vi "Day 9 - Rope Bridge.vi"() -> ()   [LabVIEW 2020, in "AoC 2022.lvlib"]
uses:
  AoC 2022.lvlib
panel:
  in  "Puzzle Input":string="R 4\nU 4\nL 3\nD 1\nR 4\nD 1\nL 5\nR 2"
  out "Puzzle Part-2 Answer":string
  out "Puzzle Answer":string
  # "Press Ctrl+M & Enter the Puzzle Input and run the VI"
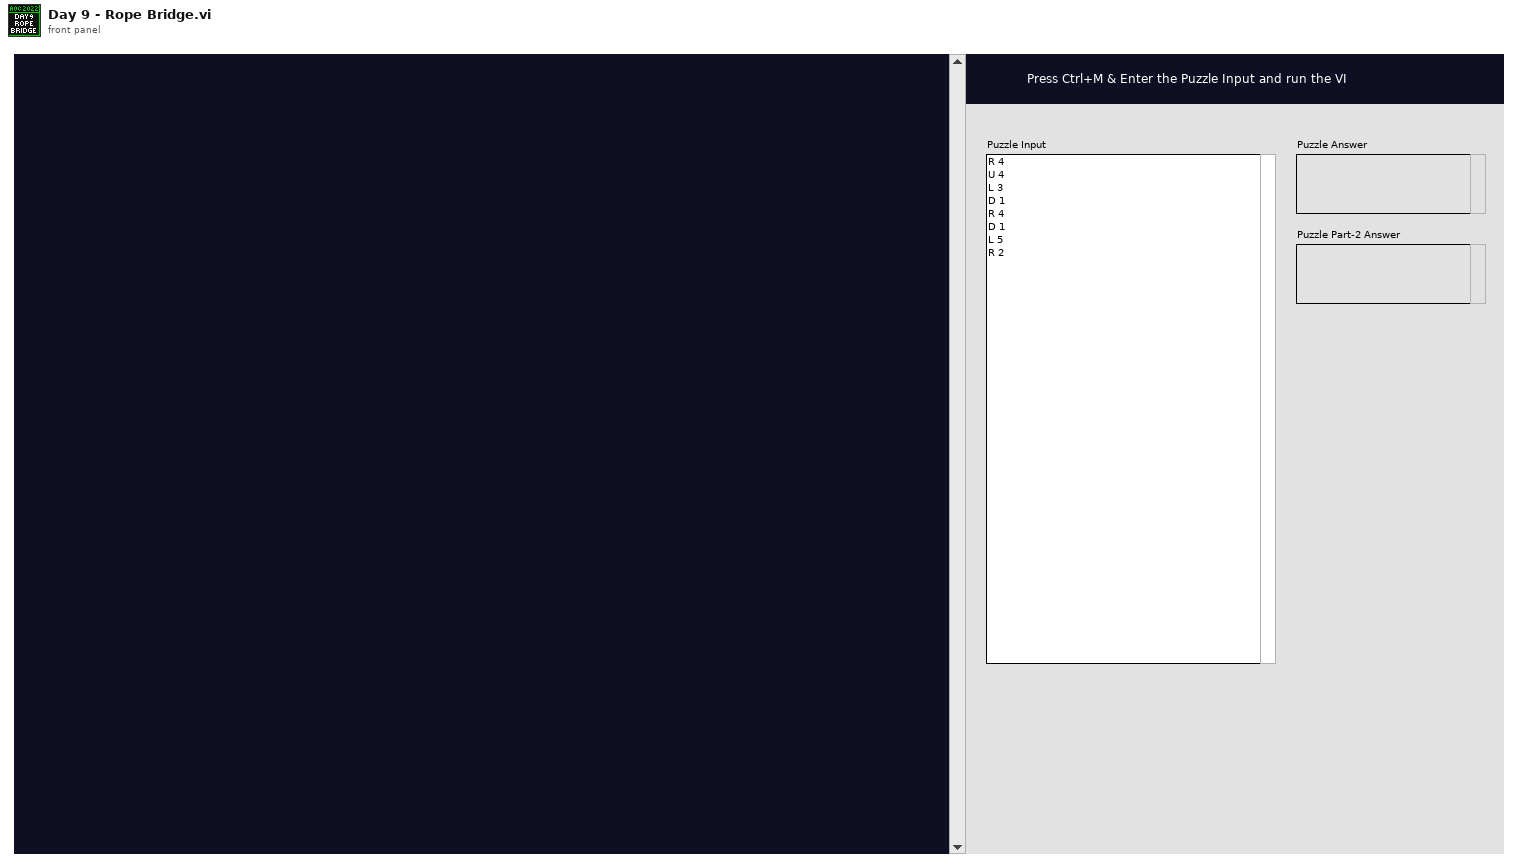
[diagram p1: front panel]
types:
  T1 = typedef "AoC 2022.lvlib/Rope Data.ctl" = map{i32, T2}
  T2 = typedef "AoC 2022.lvlib/Positions.ctl" = cluster{"H Direction":string, "H":cdb, "Knots":cdb[], "T":cdb}
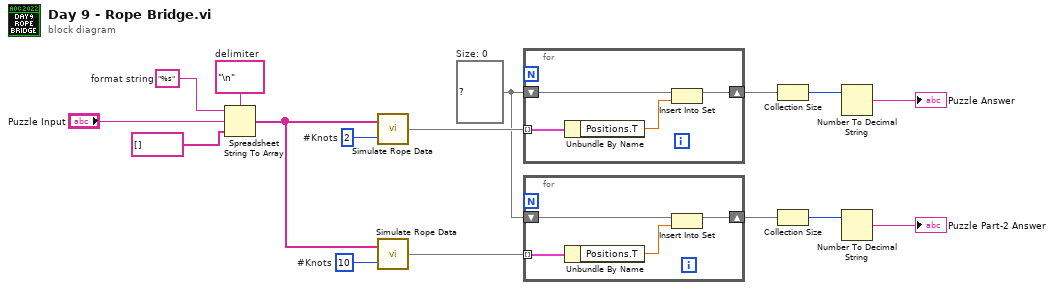
[diagram p0: block diagram]
diagram:
  w7 = 10  # #Knots
  w9 = 2  # #Knots
  w3 = set{cdb} {}  # Size: 0
  w14 = "%s"  # format string
  w16 = "\n"  # delimiter
  n1 = Spreadsheet String To Array(delimiter (Tab)=w16, format string=w14, spreadsheet string="Puzzle Input", array type (2D Dbl)=string[] []) -> (array=w8:string[])
  n2 = call "Simulate Rope Data.vi"("#Knots"=w9, "Moves"=w8) -> ("Rope Data"=w4:T1)  [unwired: 1 in]
  n3 = call "Simulate Rope Data.vi"("#Knots"=w7, "Moves"=w8) -> ("Rope Data"=w2:T1)  [unwired: 1 in]
  n4 = for {
    tunnel: w4 -> [w20] mode=indexing
    shift-right: [w18] -> w10
    shift-left: w3 -> [w17]
    n5 = Unbundle By Name(w20) -> ("Positions.T"=w19:cdb)
    n6 = Insert Into Set(10:w19, 11:w17) -> (3:w18:set{cdb})  [unwired: 1 out]
  }
  n7 = for {
    tunnel: w2 -> [w24] mode=indexing
    shift-right: [w22] -> w1
    shift-left: w3 -> [w21]
    n8 = Unbundle By Name(w24) -> ("Positions.T"=w23:cdb)
    n9 = Insert Into Set(10:w23, 11:w21) -> (3:w22:set{cdb})  [unwired: 1 out]
  }
  n10 = Collection Size(1:w10) -> (0:w12:i32)
  n11 = Collection Size(1:w1) -> (0:w6:i32)
  n12 = Number To Decimal String(number=w12) -> (decimal integer string=→"Puzzle Answer":string)  [unwired: 1 in]
  n13 = Number To Decimal String(number=w6) -> (decimal integer string=→"Puzzle Part-2 Answer":string)  [unwired: 1 in]
